vi "run.vi"(8 "error in (no error)":errorcluster, 11 "MonoCommunicator in":refnum<class "MonoCommunicator.lvclass">) -> (0 "error out":errorcluster, 3 "MonoCommunicator out":refnum<class "MonoCommunicator.lvclass">)   [LabVIEW 2016, in "MonoCommunicator.lvclass"]
uses:
  MonoCommunicator.lvclass
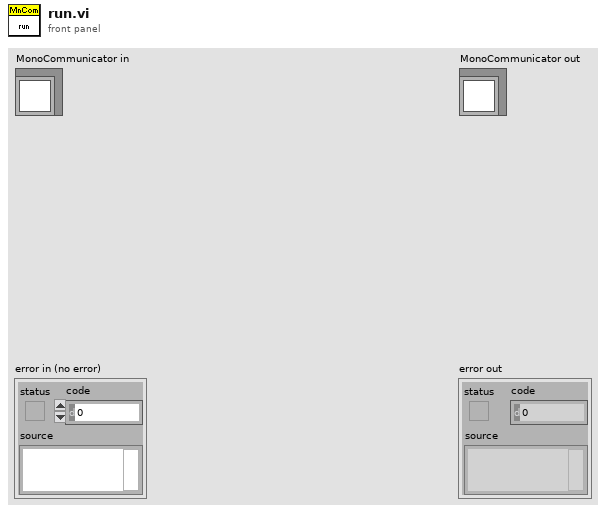
[diagram p1: front panel]
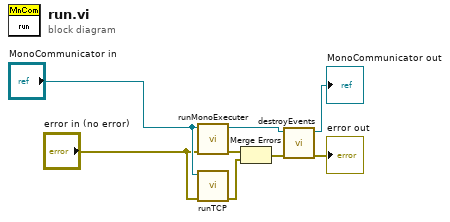
[diagram p0: block diagram]
diagram:
  n1 = call "runMonoExecuter.vi"("error in (no error)"="error in (no error)", "MonoCommunicator in"="MonoCommunicator in") -> ("error out"=w8:errorcluster, "MonoCommunicator out"=w4:refnum<class "MonoCommunicator.lvclass">)  [unwired: 8 in]
  n2 = call "runTCP.vi"("error in (no error)"="error in (no error)", "MonoCommunicator in"="MonoCommunicator in") -> ("error out"=w7:errorcluster)  [unwired: 8 in, 1 out]
  n3 = Merge Errors(w8, w7) -> (w6:errorcluster)
  n4 = call "destroyEvents.vi"("error in (no error)"=w6, "MonoCommunicator in"=w4) -> ("error out"=→"error out":errorcluster, "MonoCommunicator out"=→"MonoCommunicator out":refnum<class "MonoCommunicator.lvclass">)  [unwired: 8 in]
